vi "plateau gradient.vi"() -> ()   [LabVIEW 2016]
panel:
  out "B, mu, slope (at min)":dbl[][](array[numeric])=[[-18.0004, 0.34083294248369717, -5.173234765856728], [-17.9998, 0.35388834882623726, -6.191768731857549], [-17.8137, 0.37854792147689775, -14.547505457305519], [-17.6036, 0.40298491647823015, -18.461474456997593], [-17.394, 0.4263155355274627, -20.054679527957646], [-17.1842, 0.4493670436238973, -26.183274246034124], [-16.9746, 0.4786955891171143, -22.899459550875246], [-16.7645, 0.5008422799103762, -28.282500459765252], [-16.5563, 0.5261564535925373, -28.329338685926018], [-16.3467, 0.55558688553236, -30.880294434089127], [-16.1368, 0.5825834598122559, -33.96912211175529], [-15.9287, 0.6142937905244039, -15.967671596492483], [-15.7185, 0.6414293224999177, -20.55161222698465], [-15.5089, 0.6646469710614371, -22.358270662383717], [-15.2992, 0.690325915619735, -24.57473016416589], [-15.0895, 0.7188617607559091, -16.927574657518374], [-14.8796, 0.7396374633093362, -2.1534465442949453], [-14.67, 0.7703704058296005, -5.719879737672517], [-14.4602, 0.7865691716647003, -4.15661854433157], [-14.2521, 0.8097677713099629, -10.261898484827947], [-14.0423, 0.808252420511122, -5.0398354957743585], [-13.8327, 0.8382763751868431, -7.669659584920829], [-13.6229, 0.8494812080274252, -8.37894679879847], [-13.4133, 0.8681673037962536, -17.96741436902646], [-13.2049, 0.8765314564799321, 2.5477433740386175], [-12.9953, 0.8950037738837515, -0.02620894872773503], [-12.7852, 0.8971021344433163, -17.93838176016655], [-12.5773, 0.9085272799705543, -21.777142454045123], [-12.3674, 0.9090253438836542, -15.769540204471284], [-12.1577, 0.9156256702141738, -8.45949797995927], [-11.9476, 0.9262279968691314, -6.1806952177660905], [-11.7381, 0.9268401046719934, -5.433877749737133], [-11.5296, 0.9274941715130582, -10.558365081676799], [-11.3198, 0.9260049834958971, -3.0232237218470432], [-11.11, 0.9202154164553267, -12.789265448278176], [-10.9003, 0.9374779304631722, -12.37022006982701], [-10.6906, 0.9339958695175558, -12.363299724711608], [-10.4811, 0.9341038336467408, -2.449564789721579], [-10.2715, 0.9205103645478008, -4.26704714748349], [-10.062, 0.9194576077181751, -5.542850368649428], [-9.8526, 0.9341765353738685, -7.536919870492647], [-9.6425, 0.9246033463162676, -0.28333243847677964], [-9.4322, 0.9376682616607592, -3.167884314433153], [-9.2222, 0.9409086059748072, -8.733937361120596], [-9.0141, 0.8153719431820567, -5.878376793473805], [-8.8044, 0.9483996578275129, 5.845159510196036], [-8.5948, 0.8446703285155848, 8.883665788751491], [-8.3845, 0.9267295169496182, 21.80176168771906], [-8.1753, 0.8502501464403269, 8.98500516619147], [-7.9654, 0.8398606028004503, 1.4884008902815717], [-7.7557, 0.8171087217376165, 12.99744524005475], [-7.546, 0.8620634189234949, 22.893361026288858], [-7.3371, 0.8605811570101747, 25.432801462233368], [-7.1273, 0.7575764511858176, 25.394449007662946], [-6.9162, 0.7506662861383073, 22.881276973761164], [-6.7067, 0.7607692455891788, 35.38828871971097], [-6.4971, 0.7636403402426624, 16.836453747877105], [-6.2873, 0.7800495713234741, -8.949235890462583], [-6.0778, 0.828745792788834, -4.370516007489385], [-5.8686, 1.5966156385123205, 22.38089432127768], [-5.6592, 0.7531402705616779, 37.1555958985987], [-5.4498, 0.734101287775924, 37.57592471253709], [-5.2386, 0.7139030916248037, 25.607525065656194], [-5.0305, 0.7681397845743694, 9.155830708505334], [-4.8198, 0.8138067651617811, 3.715647239314276], [-4.6107, 0.8609652829782128, 50.69856209380314], [-4.4025, 1.2549265568153447, 59.734015181417504], [-4.1931, 1.2376859384926409, 19.25835298674846], [-3.9835, 1.2851301668781985, 6.746459524550551], [-3.7744, 1.2834061736052156, -4.969710118384977], [-3.5651, 1.3351362515582252, 37.99384843551046], [-3.3555, 1.5346196066748345, 8.69187098505985], [-3.1443, 1.3412764633999585, -2.986523762084303], [-2.9325, 1.5014452902674384, 2.3381975571350444], [-2.7262, 1.3539781217868212, 7.527042437087239], [-2.5165, 1.5478717210203718, 7.931787922509195], [-2.3062, 1.552104806368273, 26.096817100559534], [-2.0979, 1.6077226449724464, -125.36598770523698], [-1.8884, 1.5641764475436093, -29.47565227422631], [-1.6786, 1.6402722433623762, 0.10681608896589974], [-1.468, 1.6712181829109292, -61.2939953419888], [-1.2578, 1.632790698218865, 45.210940825730134], [-1.0491, 1.6329931766551624, 6.172169543990686], [-0.8365, 1.6094066360611232, -16.68977766864009], [-0.6289, 1.6342543861496224, 3.609311292837699], [-0.4182, 1.235833064309097, -22.422995366393028], [-0.2096, 1.2490647173851361, 33.5177431804831], [0.0006, 1.690674835459168, -99.84418002104957], [0.2111, 1.5985726405217648, -70.96246160014357], [0.4199, 1.5926904941220985, -75.75835421931646], [0.6277, 1.542163630678272, -70.94384920581913], [0.8368, 1.626407524228521, -2.9207757193572244], [1.0468, 1.6172800440668813, -61.15661795520781], [1.2564, 1.6550297190846754, -97.23417807267055], [1.4643, 1.6119809063266322, -30.267830153484415], [1.6748, 1.5396579552388947, -47.529715062252855], [1.8832, 1.4898748275890548, -34.95832551774146], [2.0939, 1.555000258804947, -58.9107902748855], [2.3032, 1.5094377301220825, -82.20872504623873], [2.5144, 1.4963613011056487, -17.92842607769794], [2.7237, 1.3416308852178176, -21.090299792770217], [2.9332, 1.3662322940396203, -8.763125873683537], [3.1425, 1.5195157103964436, -51.31403000485056], [3.3523, 1.5972333202906273, 6.81439969408703], [3.5631, 1.3157854155646498, -29.410781248325993], [3.7729, 1.2966361978928982, -16.128223811221268], [3.9819, 1.1852108185707344, 14.90987442582412], [4.1914, 1.6574245329762087, -32.88783257819091], [4.4021, 1.6602470071863675, 12.352768308241828], [4.6101, 1.698552024459783, 39.72592024222971], [4.8206, 1.613893664476783, -20.698266073430265], [5.0302, 1.5661369236872755, 9.191903813882345], [5.2398, 1.5317492745397208, 31.82167208780665], [5.4493, 1.7032206534536571, 27.2279812169822], [5.6584, 1.5873101218914083, -23.573587079920056], [5.8691, 0.7880587848451807, -28.309054003786], [6.0784, 1.5668965459766868, 24.465795678541877], [6.2876, 1.6647909223709836, 4.941627662907951], [6.4968, 0.9033303910526695, 24.95828093704544], [6.7057, 0.7520681016126401, 23.342335659536136], [6.9171, 0.8267635390535882, 6.983358845479114], [7.1262, 0.872693445959905, -2.6923116582484585], [7.336, 0.8069357417098988, -15.23055862298106], [7.5435, 0.8580422488112427, 5.550871789387957], [7.7545, 0.8165626488945097, -14.937956374969641], [7.9638, 0.8101163751678151, 7.954926215998341], [8.1734, 0.885368052859967, 18.474494421317544], [8.3829, 0.9519471439397811, 0.538415900652733], [8.5923, 0.8307491729897896, -3.4015856033553504], [8.802, 0.9423318953819324, -18.064264639805465], [9.0116, 0.9318653646532356, -17.354678806382292], [9.2206, 0.9141721063882297, -25.97941863813034], [9.4321, 0.9217474989496457, -9.134231346707537], [9.6403, 0.8411075667205083, -22.79982668295941], [9.8516, 0.9318079708537922, -15.21571404061835], [10.0609, 0.9353028393128109, -22.803363283235825], [10.2704, 0.9303086446891058, -11.605307683124833], [10.4793, 0.9382510660419905, -12.503621636144057], [10.6894, 0.9370909628145874, -19.662468477106305], [10.8992, 0.9301157516618346, -18.91137291654334], [11.1084, 0.9151595812379345, -8.455329151260992], [11.3181, 0.938330680761503, -22.32146964526445], [11.5275, 0.9221209575004647, -21.185824040072372], [11.7369, 0.913338000983106, -16.12971839062216], [11.9465, 0.9197912442629096, -9.489924444607833], [12.1554, 0.9089711889667003, -24.620287709336882], [12.366, 0.90658841540155, -27.277451175452946], [12.5761, 0.8846147104164821, -18.379227744069702], [12.7847, 0.8914058476816962, -28.351142283190725], [12.995, 0.8883413678596191, -28.157621703523535], [13.2052, 0.8609218051280461, -17.53494149976276], [13.4153, 0.8428925241176285, -20.762537496946894], [13.6251, 0.835772285843422, -34.28673664663465], [13.8337, 0.8180421155572588, -14.890875007105821], [14.0433, 0.8064425674146741, -36.68755595264384], [14.2535, 0.7708009172021453, -21.961802844195375], [14.4621, 0.7482984317990662, -25.838446943821914], [14.6726, 0.7276688663105734, -27.462365937618912], [14.8827, 0.7077720742079305, -44.5515368806895], [15.0929, 0.6812318114975486, -49.72881863654704], [15.3032, 0.642464685987039, -42.95657217077988], [15.5113, 0.6238252776329374, -52.33206380875328], [15.7213, 0.5879658584267555, -52.307835498127524], [15.9304, 0.5639481541009435, -57.29054416814227], [16.1402, 0.5286852951428236, -56.124796961842456], [16.349, 0.5090817673045982, -47.21072829798949], [16.559, 0.48991981193292766, -50.58927466384655], [16.7671, 0.4559185008762737, -45.62236631295394], [16.9778, 0.4327388847530754, -44.58955978695358], [17.1861, 0.4051557589898407, -35.153051608469575], [17.3978, 0.390153949471207, -34.734613585053665], [17.6064, 0.36527901433705656, -16.13423022922853], [17.8158, 0.3369284256448293, -15.62841265156498]]
  out "min slope":dbl=-4.15661854433157
  out "plateau posistion (min slope)":dbl=0.7865691716647003
  out "slope at cursor":dbl=-4.15661854433157
  out "Conductance 3":cluster{dbl[], dbl[]}[](graph)=[{[0.0005000000000000039, 0.0007500000000000041, 0.001000000000000004, 0.001250000000000005, 0.001500000000000005, 0.001750000000000005, 0.002000000000000002, 0.002250000000000002, 0.002500000000000002, 0.002750000000000002, 0.003000000000000003, 0.003250000000000003, 0.003500000000000003, 0.003750000000000003, 0.004000000000000004, 0.004250000000000004, 0.004500000000000004, 0.004750000000000004, 0.005000000000000004, 0.005250000000000005, 0.005500000000000005, 0.005750000000000005, 0.006000000000000005, 0.006250000000000002, 0.006500000000000002], [0.5871498938204003, 0.6141671925515462, 0.640109986899707, 0.6638357131505589, 0.6874438669401491, 0.7112965423731699, 0.7332514678578941, 0.7523122491420182, 0.7677129314542661, 0.7780953277698436, 0.7833065677079711, 0.7861188234413321, 0.7876618586986562, 0.7865691716647003, 0.7855835494264904, 0.7883793442369216, 0.7942784285191782, 0.8024188913587017, 0.8138845105569553, 0.8295603629368333, 0.8480658341313498, 0.866701237300026, 0.8836321919101746, 0.8982438320305886, 0.9107785923232934]}, {[0.0005000000000000039, 0.009752934579389999], [0.5871498938204003, 1.5871070845049164]}, {[0.0007500000000000041, 0.01019065028898906], [0.6141671925515462, 1.6141226286196346]}, {[0.001000000000000004, 0.011066228288873044], [0.640109986899707, 1.6400593211402157]}, {[0.001250000000000005, 0.011812668986796742], [0.6638357131505589, 1.6637799266064275]}, {[0.001500000000000005, 0.012034418886569795], [0.6874438669401491, 1.6873883784100219]}, {[0.001750000000000005, 0.012664568917440033], [0.7112965423731699, 1.7112369766918079]}, {[0.002000000000000002, 0.014189546194548746], [0.7332514678578941, 1.7331771725797855]}, {[0.002250000000000002, 0.01675743319211198], [0.7523122491420182, 1.7522070107955516]}, {[0.002500000000000002, 0.02188891843918738], [0.7677129314542661, 1.7675249487063884]}, {[0.002750000000000002, 0.03479789178509958], [0.7780953277698436, 1.7775816621597293]}, {[0.003000000000000003, 0.0651963278283812], [0.7833065677079711, 1.7813705019349646]}, {[0.003250000000000003, 0.11730375462846428], [0.7861188234413321, 1.7795934034156513]}, {[0.003500000000000003, 0.7465367780101406], [0.7876618586986562, 1.4569124444468562]}, {[0.003750000000000003, 0.23765627262905034], [0.7865691716647003, -0.18568997878068616]}, {[0.004000000000000004, 0.2702466929166942], [0.7855835494264904, 1.7494884713513261]}, {[0.004250000000000004, 0.06166026757256633], [0.7883793442369216, 1.7867300146815537]}, {[0.004500000000000004, 0.04009112080643384], [0.7942784285191782, 1.7936448638769713]}, {[0.004750000000000004, 0.030244001636673422], [0.8024188913587017, 1.8020938664783899]}, {[0.005000000000000004, 0.023418867882414086], [0.8138845105569553, 1.8137148688207612]}, {[0.005250000000000005, 0.019876306492808166], [0.8295603629368333, 1.829453392794717]}, {[0.005500000000000005, 0.018961037378306175], [0.8480658341313498, 1.8479752302631693]}, {[0.005750000000000005, 0.019806839949179353], [0.866701237300026, 1.8666024350444046]}, {[0.006000000000000005, 0.021849589989350243], [0.8836321919101746, 1.8835065792694916]}, {[0.006250000000000002, 0.02466552479571749], [0.8982438320305886, 1.8980742518751232]}, {[0.006500000000000002, 0.02644057213056871], [0.9107785923232934, 1.91057975934757]}]
  out "Slope Unit Vector[x,y,slope] 2":dbl[][](array[numeric])=[[0.009252934579389995, 0.999957190684516, 108.06919492458347], [0.009440650288989057, 0.9999554360680886, 105.92018615861342], [0.01006622828887304, 0.9999493342405086, 99.33704119802528], [0.010562668986796737, 0.9999442134558685, 94.6677600808841], [0.01053441888656979, 0.9999445114698727, 94.92165844522194], [0.010914568917440028, 0.999940434318638, 91.61520183549038], [0.012189546194548744, 0.9999257047218914, 82.03141353769722], [0.01450743319211198, 0.9998947616535334, 68.92292719274413], [0.01938891843918738, 0.9998120172521224, 51.56615725565072], [0.03204789178509958, 0.9994863343898858, 31.187272507409965], [0.062196327828381186, 0.9980639342269935, 16.046991342977016], [0.11405375462846427, 0.9934745799743192, 8.710581981370202], [0.7430367780101407, 0.6692505857482001, 0.9006964467364041], [0.23390627262905034, -0.9722591504453865, -4.15661854433157], [0.26624669291669417, 0.9639049219248357, 3.620345144442532], [0.05741026757256633, 0.9983506704446321, 17.389758185375484], [0.03559112080643383, 0.999366435357793, 28.079094243560235], [0.025494001636673418, 0.9996749751196882, 39.21216407555431], [0.01841886788241408, 0.9998303582638057, 54.282943156263215], [0.01462630649280816, 0.9998930298578836, 68.36264714878885], [0.01346103737830617, 0.9999093961318194, 74.28174872638532], [0.014056839949179348, 0.9999011977443786, 71.13271555764949], [0.015849589989350238, 0.999874387359317, 63.085189461125445], [0.018415524795717488, 0.9998304198445346, 54.29280082623789], [0.01994057213056871, 0.9998011670242767, 50.13904117081931]]
  out "Slope Unit Vector[] at cursor":dbl[](array[numeric])=[0.23390627262905034, -0.9722591504453865]
  in  "length":i32=25
  in  "index 2":i32=82
  out "B":dbl=-14.4602
  in  "B field array":dbl[](array[numeric])=[-18.0004, -17.9998, -17.8137, -17.6036, -17.394, -17.1842, -16.9746, -16.7645, -16.5563, -16.3467, -16.1368, -15.9287, -15.7185, -15.5089, -15.2992, -15.0895, -14.8796, -14.67, -14.4602, -14.2521, -14.0423, -13.8327, -13.6229, -13.4133, -13.2049, -12.9953, -12.7852, -12.5773, -12.3674, -12.1577, -11.9476, -11.7381, -11.5296, -11.3198, -11.11, -10.9003, -10.6906, -10.4811, -10.2715, -10.062, -9.8526, -9.6425, -9.4322, -9.2222, -9.0141, -8.8044, -8.5948, -8.3845, -8.1753, -7.9654, -7.7557, -7.546, -7.3371, -7.1273, -6.9162, -6.7067, -6.4971, -6.2873, -6.0778, -5.8686, -5.6592, -5.4498, -5.2386, -5.0305, -4.8198, -4.6107, -4.4025, -4.1931, -3.9835, -3.7744, -3.5651, -3.3555, -3.1443, -2.9325, -2.7262, -2.5165, -2.3062, -2.0979, -1.8884, -1.6786, -1.468, -1.2578, -1.0491, -0.8365, -0.6289, -0.4182, -0.2096, 0.0006, 0.2111, 0.4199, 0.6277, 0.8368, 1.0468, 1.2564, 1.4643, 1.6748, 1.8832, 2.0939, 2.3032, 2.5144, 2.7237, 2.9332, 3.1425, 3.3523, 3.5631, 3.7729, 3.9819, 4.1914, 4.4021, 4.6101, 4.8206, 5.0302, 5.2398, 5.4493, 5.6584, 5.8691, 6.0784, 6.2876, 6.4968, 6.7057, 6.9171, 7.1262, 7.336, 7.5435, 7.7545, 7.9638, 8.1734, 8.3829, 8.5923, 8.802, 9.0116, 9.2206, 9.4321, 9.6403, 9.8516, 10.0609, 10.2704, 10.4793, 10.6894, 10.8992, 11.1084, 11.3181, 11.5275, 11.7369, 11.9465, 12.1554, 12.366, 12.5761, 12.7847, 12.995, 13.2052, 13.4153, 13.6251, 13.8337, 14.0433, 14.2535, 14.4621, 14.6726, 14.8827, 15.0929, 15.3032, 15.5113, 15.7213, 15.9304, 16.1402, 16.349, 16.559, 16.7671, 16.9778, 17.1861, 17.3978, 17.6064, 17.8158]
  out "Transconductance 2":cluster{"Vfast":dbl[], "Decimated Array":dbl[]}(graph)={"Vfast"=[0.001500000000000005, 0.001750000000000005, 0.002000000000000002, 0.002250000000000002, 0.002500000000000002, 0.002750000000000002, 0.003000000000000003, 0.003250000000000003, 0.003500000000000003, 0.003750000000000003, 0.004000000000000004, 0.004250000000000004, 0.004500000000000004, 0.004750000000000004, 0.005000000000000004, 0.005250000000000005, 0.005500000000000005, 0.005750000000000005, 0.006000000000000005, 0.006250000000000002, 0.006500000000000002, 0.006750000000000003, 0.007000000000000003, 0.007250000000000003, 0.007500000000000003], "Decimated Array"=[94.70122304728812, 88.94911538503068, 81.04016903332584, 70.37443974179921, 57.176527820495124, 42.96473067662228, 29.06670906333938, 17.08057864587058, 9.211278328064024, 6.473670419599634, 8.369101205756841, 14.003263737306352, 23.155777819399766, 35.00079364847002, 46.83655652562395, 56.26193611023099, 62.41809422671242, 64.81740020043054, 62.82930163260553, 56.86997016465618, 48.833162024703206, 40.46490294906271, 32.35979932473543, 24.361441240980756, 16.932825191829714]}
  out "Conductance 2":cluster{dbl[], dbl[]}[](graph)=[{[0.0005000000000000039, 0.0007500000000000041, 0.001000000000000004, 0.001250000000000005, 0.001500000000000005, 0.001750000000000005, 0.002000000000000002, 0.002250000000000002, 0.002500000000000002, 0.002750000000000002, 0.003000000000000003, 0.003250000000000003, 0.003500000000000003, 0.003750000000000003, 0.004000000000000004, 0.004250000000000004, 0.004500000000000004, 0.004750000000000004, 0.005000000000000004, 0.005250000000000005, 0.005500000000000005, 0.005750000000000005, 0.006000000000000005, 0.006250000000000002, 0.006500000000000002], [0.5871498938204003, 0.6141671925515462, 0.640109986899707, 0.6638357131505589, 0.6874438669401491, 0.7112965423731699, 0.7332514678578941, 0.7523122491420182, 0.7677129314542661, 0.7780953277698436, 0.7833065677079711, 0.7861188234413321, 0.7876618586986562, 0.7865691716647003, 0.7855835494264904, 0.7883793442369216, 0.7942784285191782, 0.8024188913587017, 0.8138845105569553, 0.8295603629368333, 0.8480658341313498, 0.866701237300026, 0.8836321919101746, 0.8982438320305886, 0.9107785923232934]}, {[0.003750000000000003, 0.23765627262905034], [0.7865691716647003, -0.18568997878068616]}]
  in  "index":i32=18
  in  "Transconductance":T1(graph)
  in  "Conductance":T1(graph)
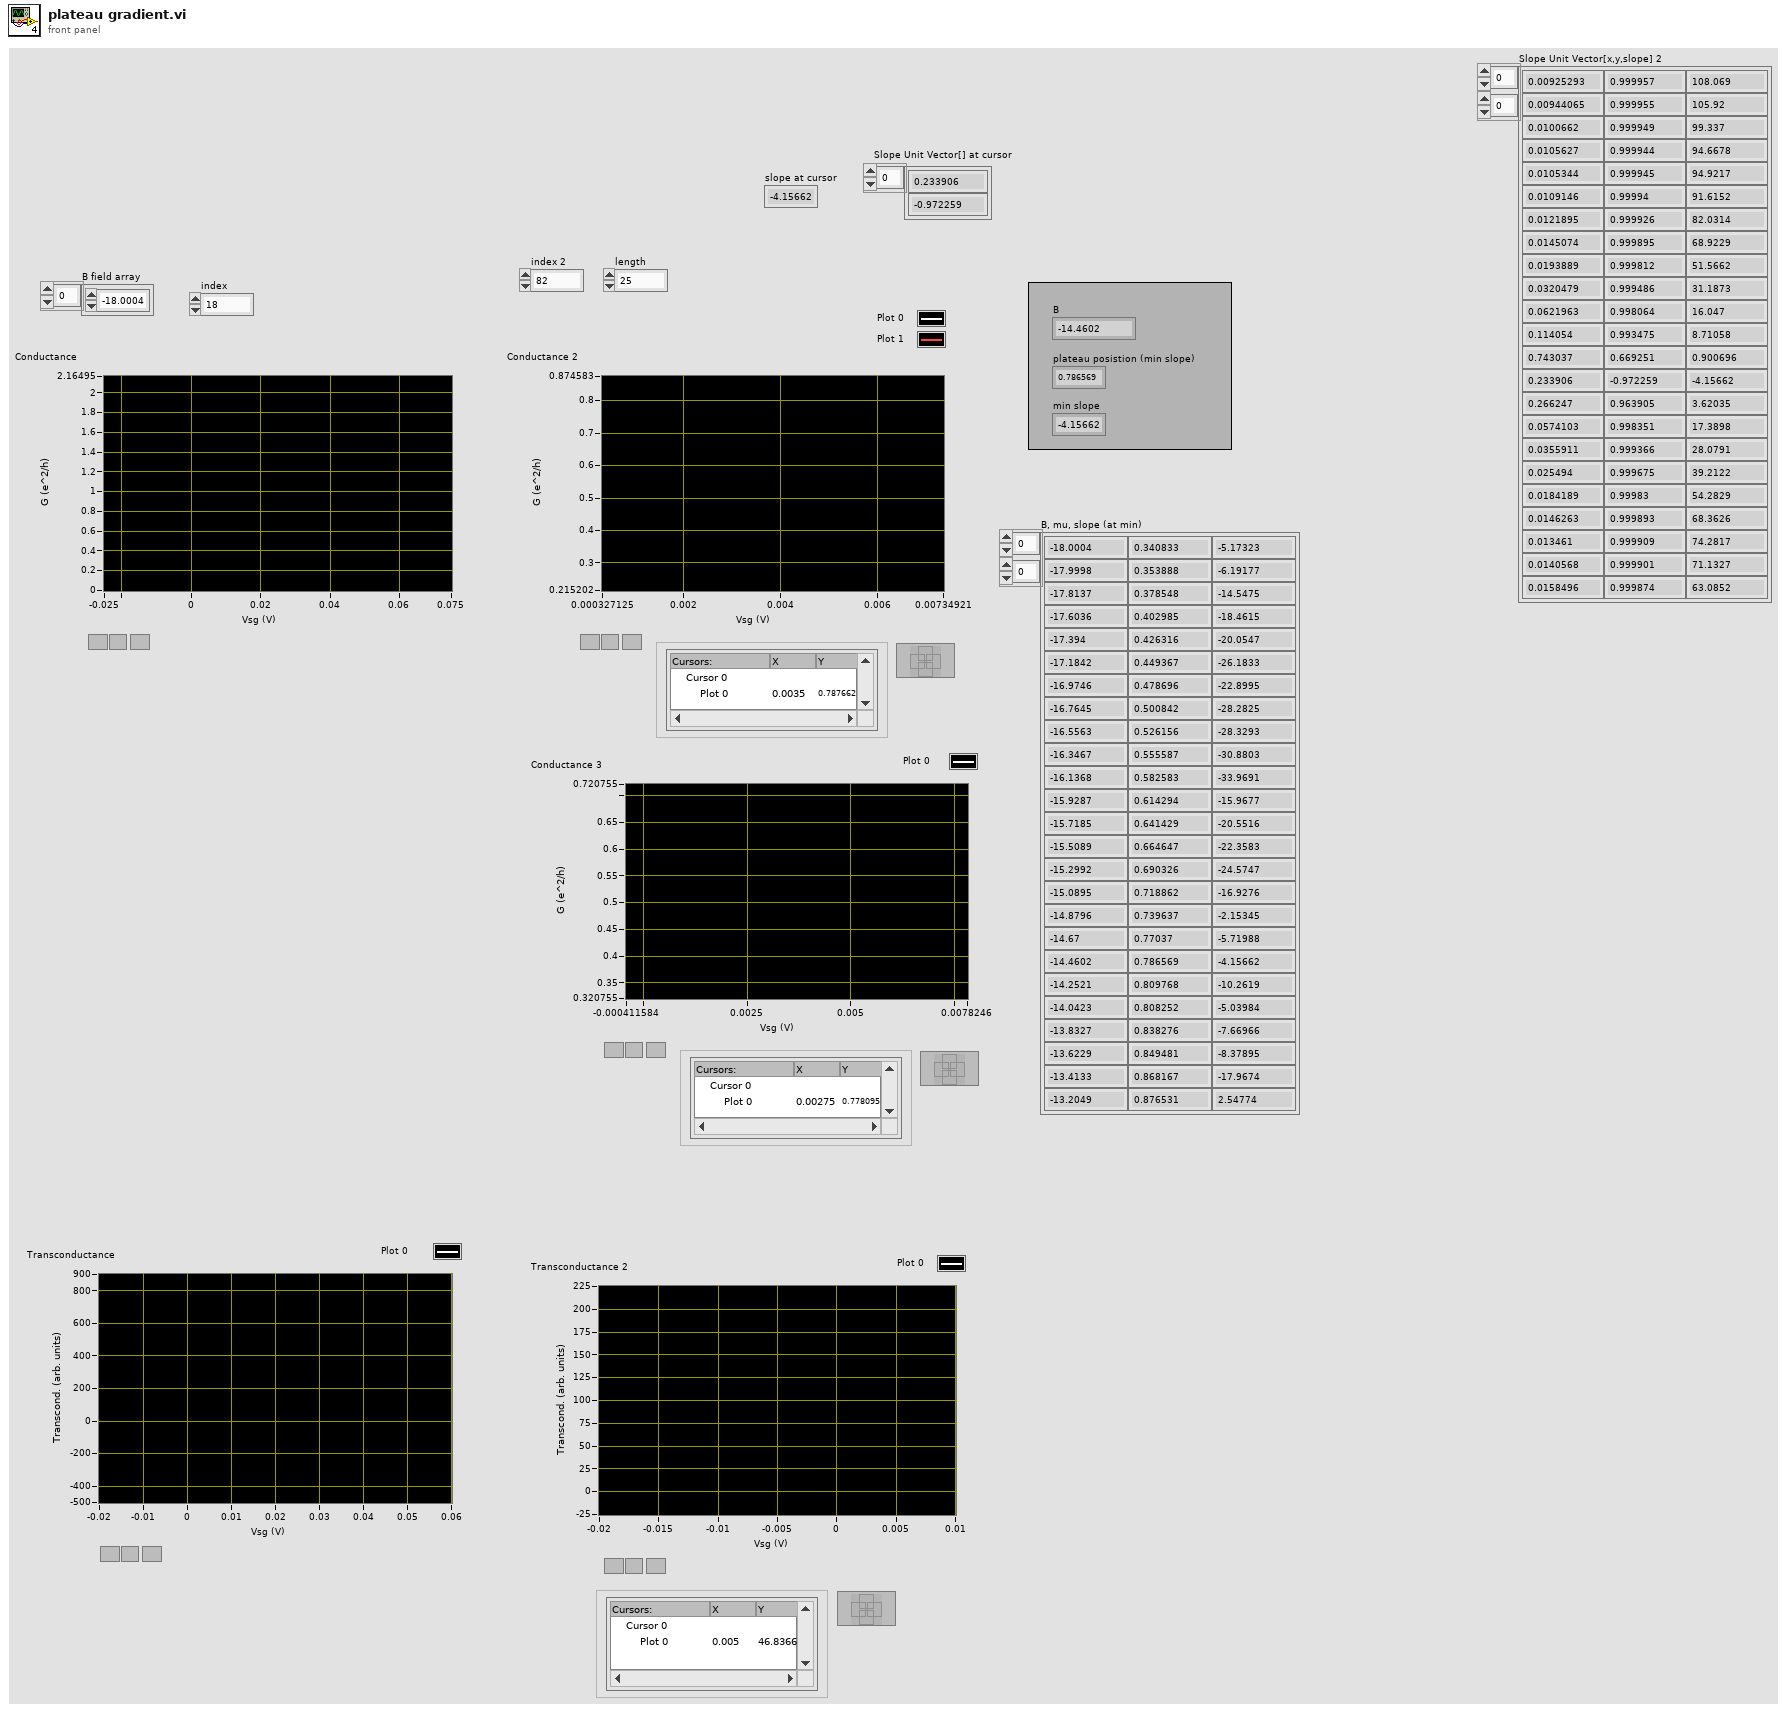
[diagram p1: front panel]
types:
  T1 = cluster{"Vfast":dbl[], "Decimated Array":dbl[]}[]
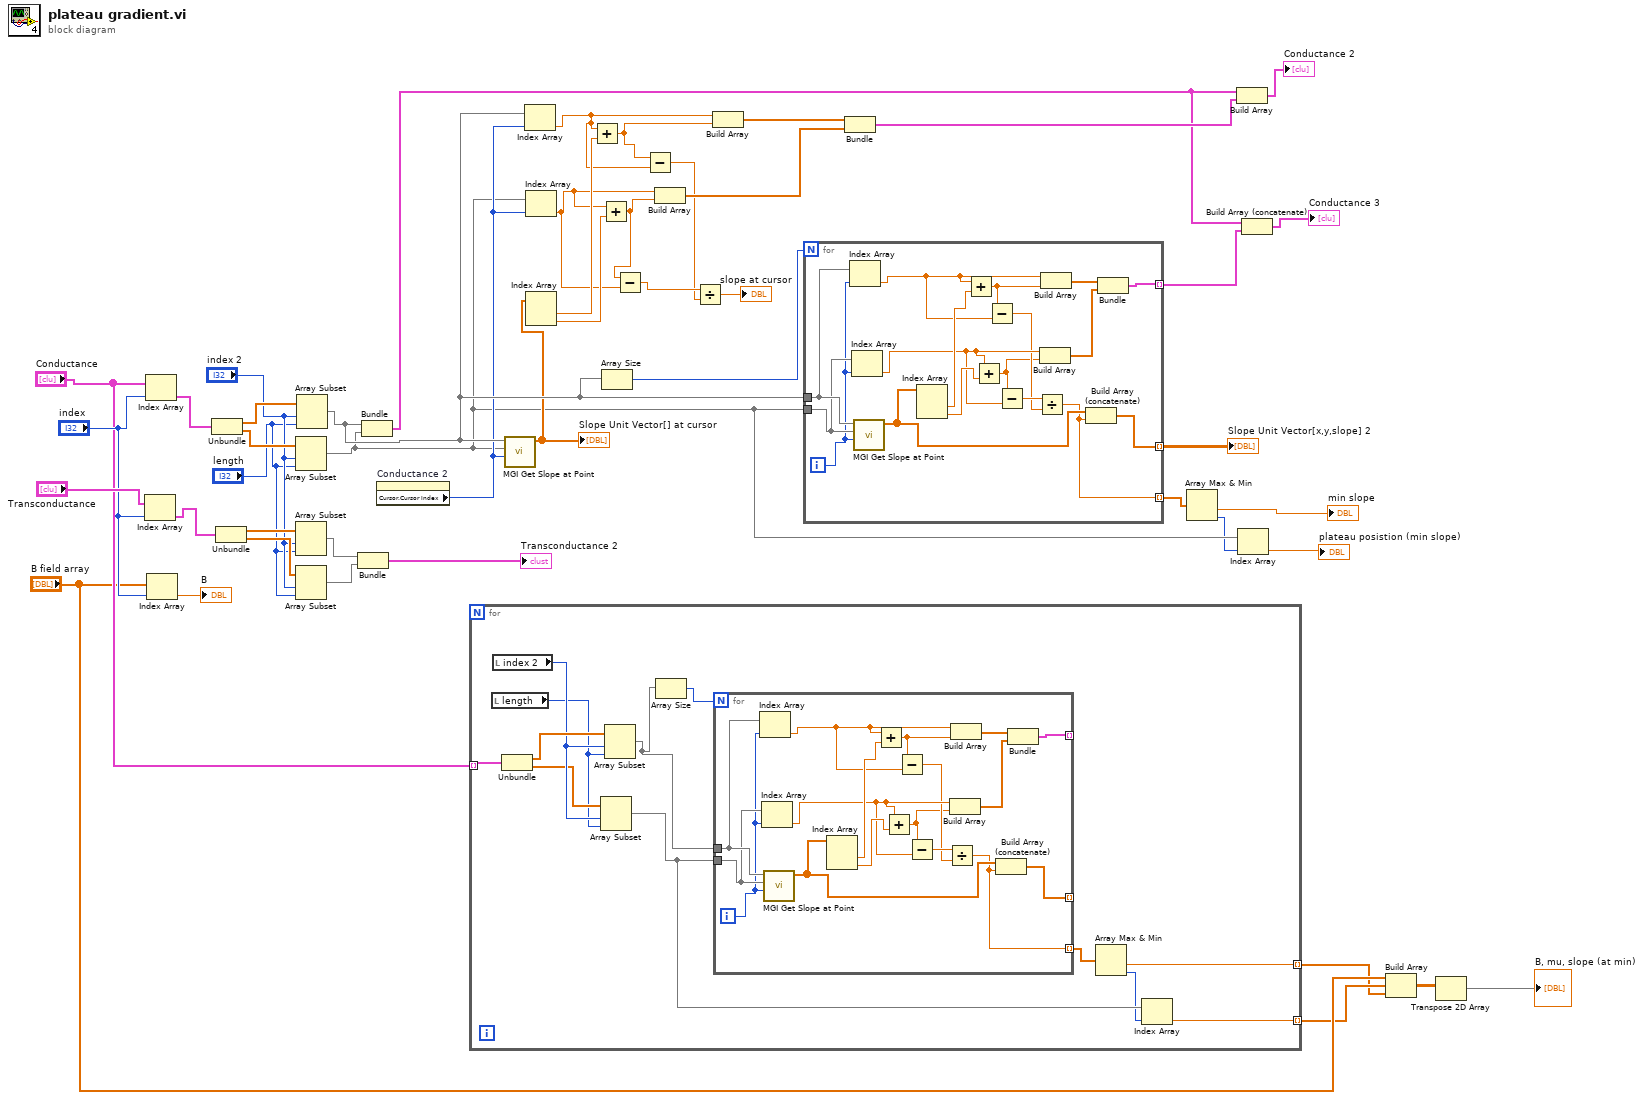
[diagram p0: block diagram]
diagram:
  n1 = Index Array(array="Transconductance", index="index") -> (element=w42:cluster{"Vfast":dbl[], "Decimated Array":dbl[]})
  n2 = Index Array(array="Conductance", index="index") -> (element=w43:cluster{"Vfast":dbl[], "Decimated Array":dbl[]})
  n3 = Index Array(array="B field array", index="index") -> (element=→"B":dbl)
  n4 = Unbundle(w43) -> ("Vfast"=w41:dbl[], "Decimated Array"=w40:dbl[])
  n5 = Unbundle(w42) -> ("Vfast"=w39:dbl[], "Decimated Array"=w38:dbl[])
  n6 = Array Subset(array=w40, index="index 2", length="length") -> (w10:dbl[])
  n7 = Array Subset(array=w39, index="index 2", length="length") -> (w35:dbl[])
  n8 = Array Subset(array=w38, index="index 2", length="length") -> (w34:dbl[])
  n9 = Array Subset(array=w41, index="index 2", length="length") -> (w29:dbl[])
  n10 = Bundle(w35, w34) -> (→"Transconductance 2":cluster{dbl[], dbl[]})  [unwired: 1 in]
  n11 = Bundle(w29, w10) -> (w23:cluster{dbl[], dbl[]})  [unwired: 1 in]
  n12 = property on="Conductance 2" class="XYGraph (strict)"() -> ("Cursor.Cursor Index"=w28:i32)  [unwired: 2 in, 2 out]
  n13 = for {
    tunnel: "Conductance" -> [w58] mode=indexing
    tunnel: [w50] -> w3 mode=indexing
    tunnel: [w49] -> w4 mode=indexing
    n14 = local read "length"() -> (w54:i32)
    n15 = local read "index 2"() -> (w56:i32)
    n16 = Unbundle(w58) -> ("Vfast"=w57:dbl[], "Decimated Array"=w55:dbl[])
    n17 = Array Subset(array=w55, index=w56, length=w54) -> (w52:dbl[])
    n18 = Array Subset(array=w57, index=w56, length=w54) -> (w48:dbl[])
    n19 = Array Size(array=w48) -> (size(s)=w47:i32)
    n20 = for {
      N: w47 -> [_]
      tunnel: w48 -> [w75]
      tunnel: w52 -> [w74]
      tunnel: [w62] -> _ mode=indexing
      tunnel: [w70] -> _ mode=indexing
      tunnel: [w59] -> w53 mode=indexing
      i -> [w73]
      n21 = Index Array(array=w75, index=w73) -> (element=w68:dbl)
      n22 = Index Array(array=w74, index=w73) -> (element=w66:dbl)
      n23 = call <userlib>:"MGI Get Slope at Point.vi"("Index"=w73, "Y[]"=w74, "X[]"=w75) -> ("Slope Unit Vector[]"=w63:dbl[])  [unwired: 8 in]
      n24 = Index Array(array=w63) -> (element #1=w69:dbl, element #2=w67:dbl)  [unwired: 2 in]
      n25 = Add(x=w68, y=w69) -> (x+y=w61:dbl)
      n26 = Add(x=w66, y=w67) -> (x+y=w60:dbl)
      n27 = Subtract(x=w61, y=w68) -> (x-y=w64:dbl)
      n28 = Subtract(x=w60, y=w66) -> (x-y=w65:dbl)
      n29 = Divide(x=w65, y=w64) -> (x/y=w59:dbl)
      n30 = Build Array(w66, w60) -> (w71:dbl[])
      n31 = Build Array(w68, w61) -> (w72:dbl[])
      n32 = Build Array (concatenate)(w63, w59) -> (w62:dbl[])
      n33 = Bundle(w72, w71) -> (w70:cluster{dbl[], dbl[]})  [unwired: 1 in]
    }
    n34 = Array Max & Min(array=w53) -> (min value=w50:dbl, min index (indices)=w51:i32)  [unwired: 2 out]
    n35 = Index Array(array=w52, index=w51) -> (element=w49:dbl)
  }
  n36 = call <userlib>:"MGI Get Slope at Point.vi"("Index"=w28, "Y[]"=w10, "X[]"=w29) -> ("Slope Unit Vector[]"=w27:dbl[])  [unwired: 8 in]
  "Slope Unit Vector[] at cursor" <- w27
  n37 = Index Array(array=w29, index=w28) -> (element=w17:dbl)
  n38 = Index Array(array=w10, index=w28) -> (element=w12:dbl)
  n39 = Index Array(array=w27) -> (element #1=w18:dbl, element #2=w20:dbl)  [unwired: 2 in]
  n40 = Add(x=w17, y=w18) -> (x+y=w13:dbl)
  n41 = Add(x=w12, y=w20) -> (x+y=w14:dbl)
  n42 = Array Size(array=w29) -> (size(s)=w32:i32)
  n43 = Subtract(x=w14, y=w12) -> (x-y=w19:dbl)
  n44 = Subtract(x=w13, y=w17) -> (x-y=w16:dbl)
  n45 = Build Array(w12, w14) -> (w25:dbl[])
  n46 = Divide(x=w19, y=w16) -> (x/y=→"slope at cursor":dbl)
  n47 = Build Array(w17, w13) -> (w26:dbl[])
  n48 = for {
    N: w32 -> [_]
    tunnel: w29 -> [w92]
    tunnel: w10 -> [w91]
    tunnel: [w79] -> w31 mode=indexing
    tunnel: [w87] -> w22 mode=indexing
    tunnel: [w76] -> w11 mode=indexing
    i -> [w90]
    n49 = Index Array(array=w92, index=w90) -> (element=w85:dbl)
    n50 = Index Array(array=w91, index=w90) -> (element=w83:dbl)
    n51 = call <userlib>:"MGI Get Slope at Point.vi"("Index"=w90, "Y[]"=w91, "X[]"=w92) -> ("Slope Unit Vector[]"=w80:dbl[])  [unwired: 8 in]
    n52 = Index Array(array=w80) -> (element #1=w86:dbl, element #2=w84:dbl)  [unwired: 2 in]
    n53 = Add(x=w85, y=w86) -> (x+y=w78:dbl)
    n54 = Add(x=w83, y=w84) -> (x+y=w77:dbl)
    n55 = Subtract(x=w78, y=w85) -> (x-y=w81:dbl)
    n56 = Subtract(x=w77, y=w83) -> (x-y=w82:dbl)
    n57 = Divide(x=w82, y=w81) -> (x/y=w76:dbl)
    n58 = Build Array(w83, w77) -> (w88:dbl[])
    n59 = Build Array(w85, w78) -> (w89:dbl[])
    n60 = Build Array (concatenate)(w80, w76) -> (w79:dbl[])
    n61 = Bundle(w89, w88) -> (w87:cluster{dbl[], dbl[]})  [unwired: 1 in]
  }
  "Slope Unit Vector[x,y,slope] 2" <- w31
  n62 = Bundle(w26, w25) -> (w24:cluster{dbl[], dbl[]})  [unwired: 1 in]
  n63 = Array Max & Min(array=w11) -> (min value=→"min slope":dbl, min index (indices)=w9:i32)  [unwired: 2 out]
  n64 = Build Array(w23, w24) -> (→"Conductance 2":cluster{dbl[], dbl[]}[])
  n65 = Index Array(array=w10, index=w9) -> (element=→"plateau posistion (min slope)":dbl)
  n66 = Build Array (concatenate)(w23, w22) -> (→"Conductance 3":cluster{dbl[], dbl[]}[])
  n67 = Build Array("B field array", w4, w3) -> (w2:dbl[][])
  n68 = Transpose 2D Array(2D array=w2) -> (transposed array=→"B, mu, slope (at min)":dbl[][])
